vi "Check Read.vi"(8 "error in (no error)":errorcluster, 11 "CIFChannels in":refnum<class "CIFChannels.lvclass">) -> (0 "error out":errorcluster, 1 "Default Value":variant, 2 "Not Connected":bool, 3 "CIFChannels out":refnum<class "CIFChannels.lvclass">)   [LabVIEW 2021, in "CIFChannels.lvclass"]
uses:
  CIFChannels.lvclass
  CIFChannels.lvclass/CIFChannels.ctl
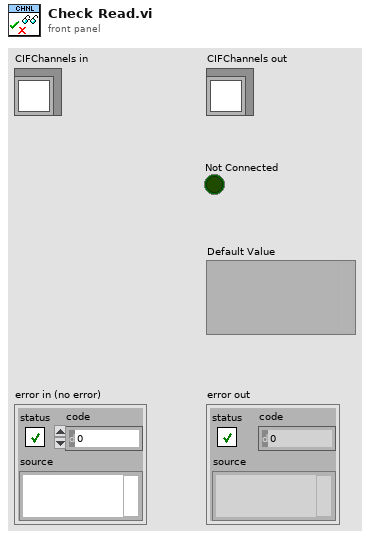
[diagram p1: front panel]
types:
  T1 = typedef "CIFChannels.lvclass/Channel State.ctl" = enum16{"Creating", "Disconnected", "Connecting", "Connected", "Destroying"}
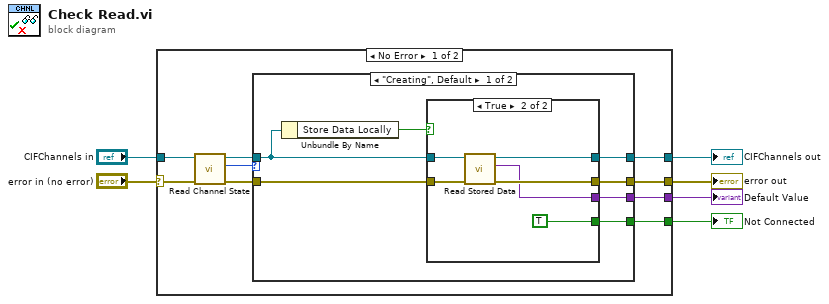
[diagram p0: block diagram]
diagram:
  n1 = case shown="No Error" "error in (no error)" {
    selector: "error in (no error)" -> [w14 w34]
    tunnel: [w7 w34] -> w5
    tunnel: [w11 w33] -> w3
    tunnel: "CIFChannels in" -> [w15 w33]
    tunnel: [w9 _] -> w2
    tunnel: [w8 _] -> w1
    frame No Error {
      n2 = call "Read Channel State.vi"("error in (no error)"=w14, "CIFChannels in"=w15) -> ("error out"=w10:errorcluster, "Channel State"=w13:T1, "CIFChannels out"=w12:refnum<class "CIFChannels.lvclass">)  [unwired: 7 in]
      n3 = case shown="\"Creating\", Default" w13 {
        tunnel: w12 -> [w20 w32]
        tunnel: [w19 w32] -> w11
        tunnel: w10 -> [w21 w31]
        tunnel: [w18 w31] -> w7
        tunnel: [w17 _] -> w9
        tunnel: [w16 _] -> w8
        frame "Creating", Default {
          n4 = Unbundle By Name(w20) -> ("Store Data Locally"=w22:bool)
          n5 = case shown="True" w22 {
            tunnel: w21 -> [w23 w29]
            tunnel: w20 -> [w24 w30]
            tunnel: [w24 w28] -> w19
            tunnel: [w23 w27] -> w18
            tunnel: [_ w26] -> w17
            tunnel: [_ TRUE] -> w16
            frame False {
            }
            frame True {
              n6 = call "Read Stored Data.vi"("error in (no error)"=w29, "CIFChannels in"=w30) -> ("error out"=w27:errorcluster, "Stored Data"=w26:variant, "CIFChannels out"=w28:refnum<class "CIFChannels.lvclass">)  [unwired: 7 in]
            }
          }
        }
        frame "Connected" {
        }
      }
    }
    frame Error {
    }
  }
  "error out" <- w5
  "CIFChannels out" <- w3
  "Default Value" <- w2
  "Not Connected" <- w1
